vi "hwOperation_Set hwName&Rate.vi"(7 "hwType":string, 8 "error in":errorcluster, 10 "Devs Info in":T1[](array[typedef]), 11 "hwDriverRef in":T3) -> (0 "error out":errorcluster, 2 "Devs Info out":T1[](array[typedef]), 3 "hwDriverRef out":T3)   [LabVIEW 2016]
uses:
  DAQ-Config/Controls/PSCHN_Card Para.ctl
  DAQ-Config/Controls/PSCHN_Channel Para.ctl
  QX/hw_QX_hwDriverRef.ctl
  C:/Users/CL/Desktop/ZcDAQprj0811/ZcDAQprj/Modules/DAQ-Device/Hardware Drivers/QX/HBM LabVIEW Driver/DLLs/Hbm.Api.Common.dll
  QX/HBM LabVIEW Driver/DLLs/Hbm.Api.Common.dll
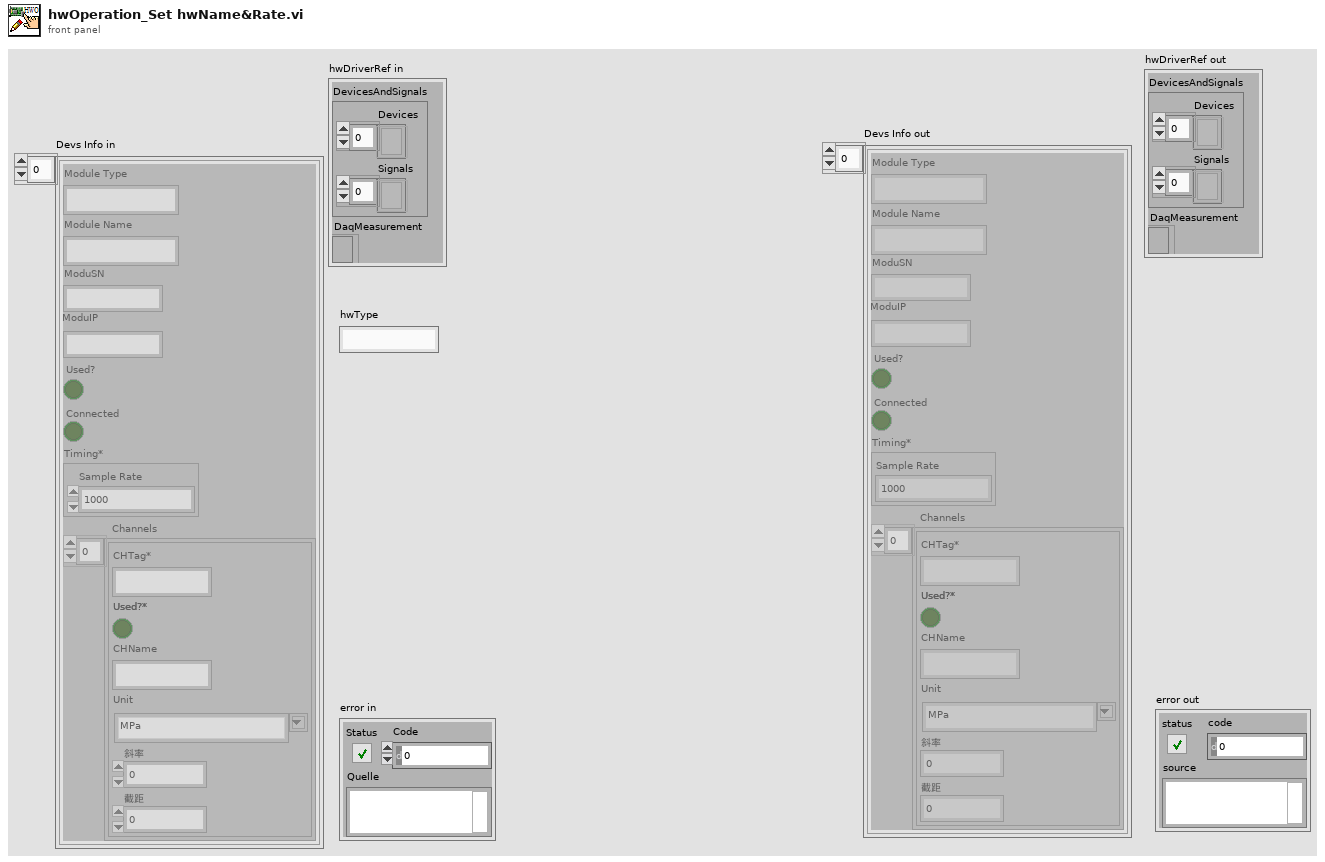
[diagram p1: front panel]
types:
  T1 = typedef "PSCHN_Card Para.ctl" = cluster{"Module Type":string, "Module Name":string, "ModuSN":string, "ModuIP":string, "Used?":bool, "Connected":bool, "Timing*":cluster{"Sample Rate":dbl}, "Channels":T2[]}
  T2 = typedef "PSCHN_Channel Para.ctl" = cluster{"CHTag*":string, "Used?*":bool, "CHName":string, "Unit":string, "斜率":dbl, "截距":dbl}
  T3 = typedef "hw_QX_hwDriverRef.ctl" = cluster{"DevicesAndSignals":cluster{"Devices":refnum<k24>[], "Signals":refnum<k24>[]}, "DaqMeasurement":refnum<k24>}
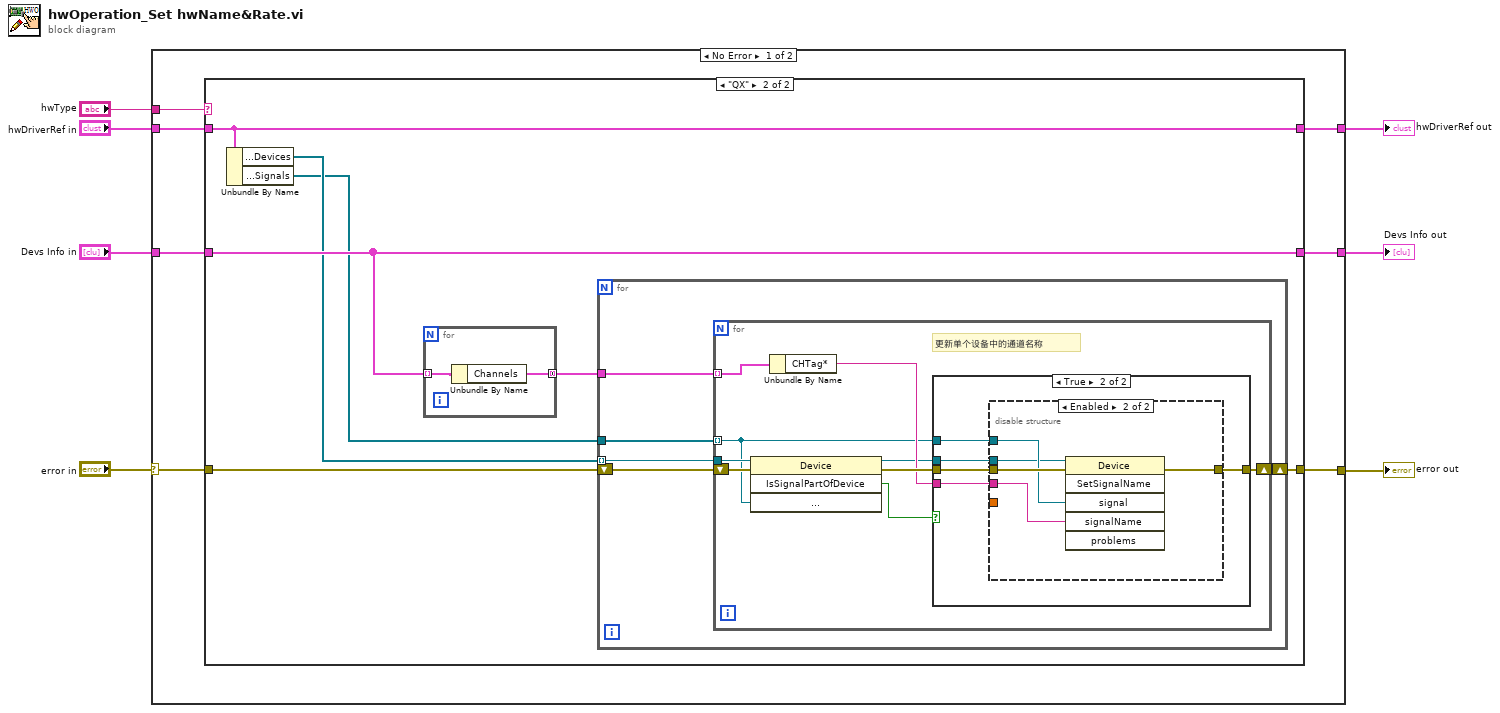
[diagram p0: block diagram]
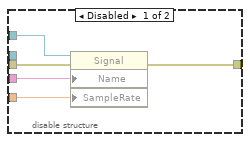
[diagram p4: hidden frame]
diagram:
  n1 = case shown="No Error" "error in" {
    selector: "error in" -> [w13 w58]
    tunnel: [w14 w58] -> w6
    tunnel: [w12 _] -> w4
    tunnel: "hwType" -> [w11 _]
    tunnel: "hwDriverRef in" -> [w10 w57]
    tunnel: [w9 w57] -> w2
    tunnel: "Devs Info in" -> [w8 _]
    frame No Error {
      n2 = case shown="\"QX\"" w11 {
        tunnel: [w17 w24] -> w14
        tunnel: w13 -> [w17 w23]
        tunnel: [w15 w22] -> w12
        tunnel: w10 -> [w16 w20]
        tunnel: [w16 w20] -> w9
        tunnel: w8 -> [w15 w22]
        frame "Simulation", Default {
        }
        frame "QX" {
          n3 = Unbundle By Name(w20) -> ("DevicesAndSignals.Devices"=w19:refnum<k24>[], "DevicesAndSignals.Signals"=w18:refnum<k24>[])
          n4 = for {
            tunnel: w22 -> [w26] mode=indexing
            tunnel: [w25] -> w21 mode=concatenating
            n5 = Unbundle By Name(w26) -> ("Channels"=w25:T2[])
          }
          n6 = for {
            tunnel: w19 -> [w29] mode=indexing
            shift-right: [w28] -> w24
            shift-left: w23 -> [w31]
            tunnel: w18 -> [w30]
            tunnel: w21 -> [w27]
            n7 = for {
              tunnel: w30 -> [w32] mode=indexing
              shift-right: [w38] -> w28
              shift-left: w31 -> [w40]
              tunnel: w29 -> [w37]
              tunnel: w27 -> [w35] mode=indexing
              # "更新单个设备中的通道名称"
              n8 = invoke on="Methodenknoten" class="Device" method="IsSignalPartOfDevice"(reference=w37, error in=w40, "signalToCheck"=w32) -> (reference out=w33:refnum<k24>, error out=w39:errorcluster, "IsSignalPartOfDevice"=w36:bool)  [unwired: 1 in, 1 out]
              n9 = Unbundle By Name(w35) -> ("CHTag*"=w34:string)
              n10 = case shown="True" w36 {
                tunnel: w39 -> [w41 w45]
                tunnel: w32 -> [_ w46]
                tunnel: [w41 w44] -> w38
                tunnel: w34 -> [_ w43]
                tunnel: w33 -> [_ w42]
                frame False {
                }
                frame True {
                  n11 = disable-structure shown="Enabled" {
                    disable-tunnel: w46 -> [w51 w54]
                    disable-tunnel: w45 -> [w50 w56]
                    disable-tunnel: [w49 w55] -> w44
                    disable-tunnel: w43 -> [w48 w52]
                    disable-tunnel: _ -> [w47 _]
                    disable-tunnel: w42 -> [_ w53]
                    frame Disabled {
                      n12 = property on="Eigenschaftsknoten" class="Signal"(reference=w51, error in=w50, "Name"=w48, "SampleRate"=w47) -> (error out=w49:errorcluster)  [unwired: 1 out]
                    }
                    frame Enabled {
                      n13 = invoke on="Methodenknoten" class="Device" method="SetSignalName"(reference=w53, error in=w56, "signal"=w54, "signalName"=w52) -> (error out=w55:errorcluster)  [unwired: 2 in, 5 out]
                    }
                  }
                }
              }
            }
          }
        }
      }
    }
    frame Error {
    }
  }
  "error out" <- w6
  "Devs Info out" <- w4
  "hwDriverRef out" <- w2
